vi "libssh2_trace_sethandler.vi"(8 "error in (no error)":errorcluster, 10 "context":refnum<user-event>, 11 "session":T1) -> (0 "error out":errorcluster)   [LabVIEW 2017, in "libssh2.lvlib"]
doc: "Set the trace handler for libssh2.\n\nThis only works on debug build of libssh2.\n\nThis function utilizes the lvssh2 extension library. You can disable the extension library by defining the LVSSH2_NO_EXTENSIONS conditional disable symbol with the value 'True' in the project properties. When the extension library is disabled, this function turns into a no-op."
uses:
  libssh2.lvlib
  Session Refnum.ctl
  Not A Session.vi
  <vilib>/Utility/error.llb/Error Cluster From Error Code.vi
  Global Settings.vi
  Read Session Refnum.vi
  <vilib>/Utility/semaphor.llb/Acquire Semaphore.vi
  <vilib>/Utility/semaphor.llb/Release Semaphore.vi
  lvssh2_extensions_64.dll
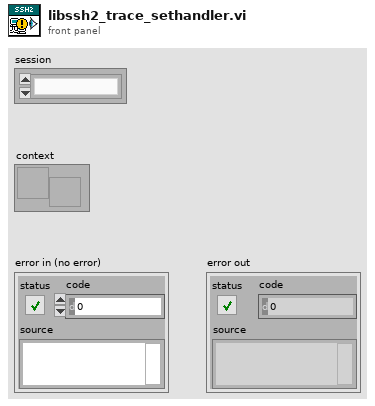
[diagram p1: front panel]
types:
  T1 = typedef "libssh2.lvlib/Session Refnum.ctl" = refnum<k1>
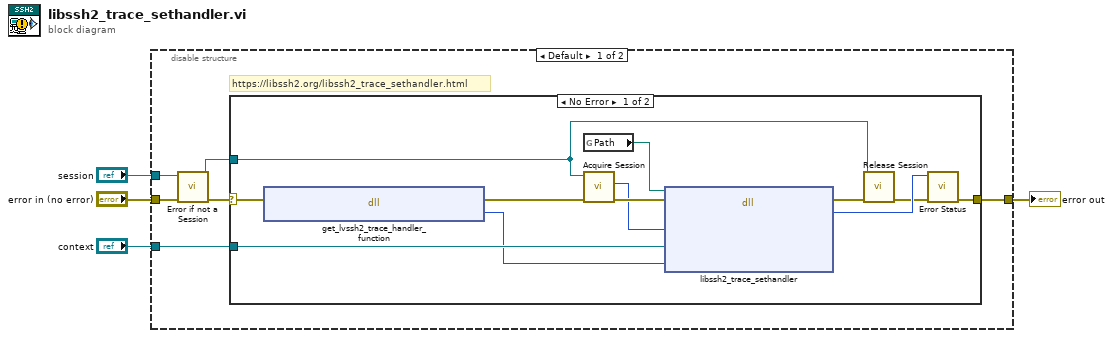
[diagram p0: block diagram]
diagram:
  n1 = disable-structure shown="Default" {
    disable-tunnel: [w10 w24] -> w4
    disable-tunnel: "error in (no error)" -> [w9 w24]
    disable-tunnel: "session" -> [w7 _]
    disable-tunnel: "context" -> [w5 _]
    frame condition #0 (active) {
      # "https://libssh2.org/libssh2_trace_sethandler.html"
      n2 = call "Error if not a Session.vi"("error in (no error)"=w9, "session"=w7) -> ("error out"=w8:errorcluster, "session out"=w6:T1)  [unwired: 8 in]
      n3 = case shown="No Error" w8 {
        selector: w8 -> [w15 w23]
        tunnel: [w22 w23] -> w10
        tunnel: w6 -> [w11 _]
        tunnel: w5 -> [w16 _]
        frame No Error {
          n4 = dll-call lib="C:/Users/pasca/Projects/Home/lvssh2/libssh2/lvssh2_extensions**.*" fn="get_lvssh2_trace_handler_function"(error in=w15) -> (error out=w14:errorcluster, "return type"=w13:u64)  [unwired: 2 in, 1 out]
          n5 = global read "Global Settings.vi" "Path"() -> (w18:path)
          n6 = call "Acquire Session.vi"("error in (no error)"=w14, "session"=w11) -> ("error out"=w20:errorcluster, "LIBSSH2_SESSION*"=w19:u64)  [unwired: 7 in, 1 out]
          n7 = dll-call lib="?" fn="libssh2_trace_sethandler"(path in=w18, error in=w20, "session"=w19, "context"=w16, "callback"=w13) -> (error out=w21:errorcluster, "return value"=w17:i32)  [unwired: 4 in, 1 out]
          n8 = call "Release Session.vi"("error in (no error)"=w21, "session"=w11) -> ("error out"=w12:errorcluster)  [unwired: 9 in]
          n9 = call "Error Status.vi"("error in (no error)"=w12, "return value"=w17) -> ("error out"=w22:errorcluster)  [unwired: 8 in, 1 out]
        }
        frame Error {
        }
      }
    }
    frame condition #1 {
    }
  }
  "error out" <- w4
